vi "Main Program Oringin.vi"() -> ()   [LabVIEW 2019]
uses:
  <vilib>/rvi/interface/nirviMethod/nirviMethod.xnode
  <vilib>/rvi/interface/nirviReadWriteControl/nirviReadWriteControl.xnode
  <vilib>/FPGAPlugInAG/Dynamic/niLvFpga_Run_Dynamic.vi
  <vilib>/FPGAPlugInAG/Dynamic/niLvFpga_Abort_Dynamic.vi
  <vilib>/platform/TimedLoop/XDataNode/XDataNode.xnode
  <vilib>/Platform/TimedLoop/XDataNode/nitl_modes.ctl
  <vilib>/Platform/TimedLoop/XDataNode/XDNodeRunTimeDep.lvlib
  <vilib>/Platform/TimedLoop/XDataNode/wakeup.ctl
  <vilib>/Platform/TimedLoop/XDataNode/timing_clust.ctl
  <vilib>/Utility/error.llb/Error Cluster From Error Code.vi
  <vilib>/rvi/interface/Simulation/niFpgaSimulationCallBeginRW.vi
  <vilib>/rvi/errors/niLvFpgaAdjustHostInterfaceError.vi
  NiFpgaLv.dll
  <vilib>/rvi/interface/nirviOpenFPGA/nirviOpenFPGA.xnode
  FPGA Bitfiles/fpgaproject_FPGATarget_Fpga_-EhYRlmx2hw.lvbitx
  Fpga.vi
  <vilib>/FPGAPlugInAG/Dynamic/niLvFpga_StartFifo_Dynamic.vi
  <vilib>/rvi/errors/niLvFpgaMergeErrorWithErrorCode.vi
  <vilib>/FPGAPlugInAG/cRIO-9065/niLvFpga_Open_cRIO-9065.vi
  <vilib>/rvi/interface/common/dynamic/niFpgaDynamicAddResources.vi
panel:
  out "error out 3":errorcluster
  in  "string":string
  in  "Vlotage In":fxp<+/-,20,5>
  out "Real Period":u32[](array[numeric])
  out "Set period":i64[](array[numeric])
  out "Real Period":u32
  out "Voltage Out":fxp<+/-,20,5>
  out "size(s)":i32[](array[numeric])
  in  "Period":i64
  out "Encoder Position":dbl format="%#_8g"
  in  "Position Reset":bool
  out "data":string[][](array[string])
  out "速率":dbl
  out "error out 2":errorcluster
  out "error out":errorcluster
  in  "stop":bool
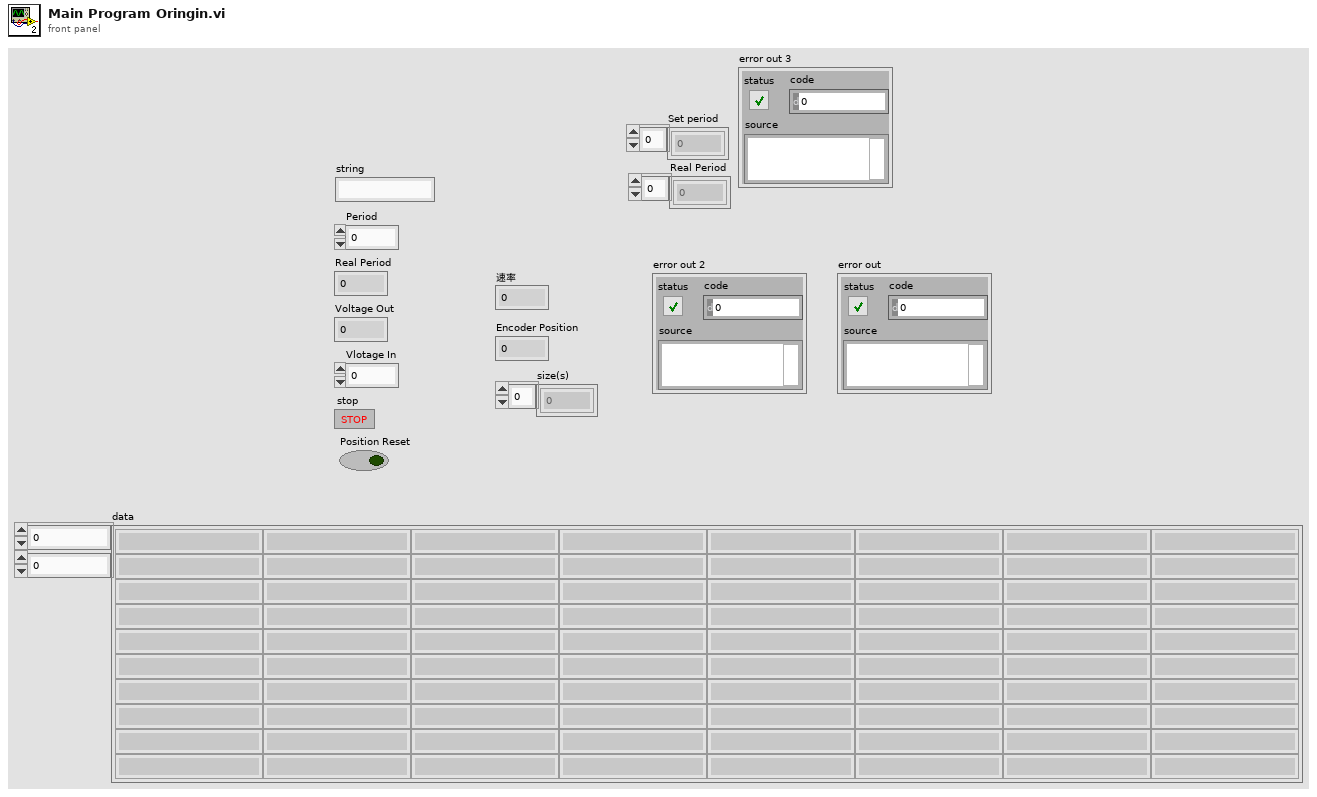
[diagram p1: front panel]
types:
  T1 = enum16{"open", "replace", "create", "open or create", "replace or create", "replace or create with confirmation"}
  T2 = typedef "XDNodeRunTimeDep.lvlib/timing_clust.ctl" = cluster{"Expected End [f-1]":u64, "Actual End [f-1]":u64, "Finished Late? [f-1]":bool, "Expected End [i-1]":u64, "Actual End [i-1]":u64, "Finished Late? [i-1]":bool, "Expected Start [i]":u64, "Actual Start [i]":u64, "Expected Start [f]":u64, "Actual Start [f]":u64, "Source Name":string, "Structure Name":string, "Period":i64, "Deadline":i64, "Offset":i64, "Start":i64, "Priority":i32, "Timeout":i32, "Mode":T3, "Wakeup Reason":T4, "Error":errorcluster, "Source Type":string, "Secondary Source Type":string, "Global End Time":u64, "Global Start Time":u64, "Frame Duration":u64, "Iteration Duration":u64, "Assigned CPU":i32, "I/O Scan Engine Mode":u32}
  T3 = typedef "XDNodeRunTimeDep.lvlib/nitl_modes.ctl" = enum32{"No Change", "Process missed periods, maintain original phase", "Discard missed periods, maintain original phase", "Process missed periods, ignore original phase", "Discard missed periods, ignore original phase"}
  T4 = typedef "XDNodeRunTimeDep.lvlib/wakeup.ctl" = enum32{"Normal", "Aborted", "Asynchronous wakeup", "Timing source error", "Timed loop error", "Timeout"}
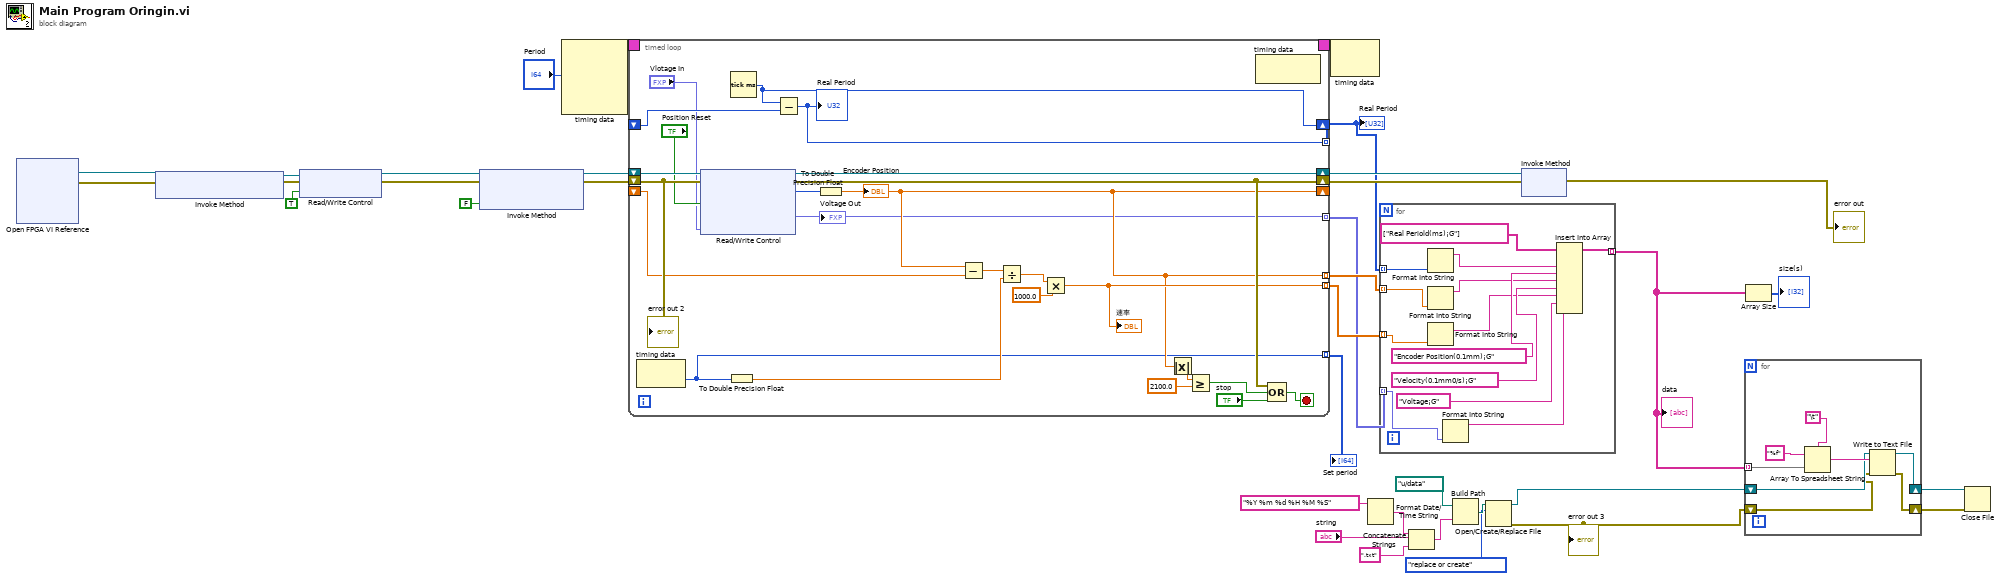
[diagram p0: block diagram]
diagram:
  n1 = xnode "Open FPGA VI Reference"() -> ("FPGA VI Reference Out"=w16:refnum<k20>, "error out"=w15:errorcluster)  [unwired: 2 in]
  n2 = xnode "Invoke Method"("FPGA VI Reference In"=w16, "error in"=w15) -> ("FPGA VI Reference Out"=w25:refnum<k20>, "error out"=w24:errorcluster)
  n3 = xnode "Read/Write Control"("FPGA VI Reference In"=w25, "error in"=w24, "Position Reset"=TRUE) -> ("FPGA VI Reference Out"=w33:refnum<k20>, "error out"=w32:errorcluster)
  n4 = xnode "Invoke Method"("FPGA VI Reference In"=w33, "error in"=w32, "Wait Until Done (F)"=FALSE) -> ("FPGA VI Reference Out"=w12:refnum<k20>, "error out"=w11:errorcluster)
  n5 = node-c288("Period") -> (w28:T2)  [unwired: 3 in]
  n6 = timed-loop {
    shift-right: [w57] -> w35
    shift-left: w12 -> [w55]
    shift-right: [w50] -> w34
    shift-left: w11 -> [w58]
    timing: w28 -> [_]
    timing-out: [_] -> w27
    shift-right: [w42] -> _
    shift-left: _ -> [w56]
    tunnel: [w42] -> w23 mode=indexing
    tunnel: [w44] -> w21 mode=indexing
    tunnel: [w41] -> w17 mode=indexing
    tunnel: [w40] -> w14 mode=indexing
    shift-right: [w38] -> _
    shift-left: _ -> [w39]
    tunnel: [w37] -> w13 mode=indexing
    stop <- w52 stop-if-true
    n7 = node-c288() -> (w40:i64)  [unwired: 1 in]
    n8 = xnode "Read/Write Control"("FPGA VI Reference In"=w55, "error in"=w58, "Position Reset"="Position Reset", "Voltage In"="Vlotage In") -> ("FPGA VI Reference Out"=w57:refnum<k20>, "error out"=w50:errorcluster, "Position (Counts)"=w47:i32, "Voltage Out"=w41:fxp<+/-,20,5>)
    "Voltage Out" <- w41
    n9 = To Double Precision Float(number=w40) -> (double precision float=w46:dbl)
    n10 = Tick Count (ms)() -> (millisecond timer value=w38:u32)
    n11 = Subtract(x=w38, y=w39) -> (x-y=w37:u32)
    "Real Period" <- w37
    n12 = To Double Precision Float(number=w47) -> (double precision float=w42:dbl)
    "Encoder Position" <- w42
    n13 = Subtract(x=w42, y=w56) -> (x-y=w59:dbl)
    n14 = Divide(x=w59, y=w46) -> (x/y=w45:dbl)
    n15 = Multiply(x=w45, y=1000.0) -> (x*y=w44:dbl)
    "速率" <- w44
    n16 = Absolute Value(x=w42) -> (abs(x)=w43:dbl)
    n17 = Greater Or Equal?(x=w43, y=2100.0) -> (x >= y?=w49:bool)
    n18 = node-c288() -> ()  [unwired: 1 in, 1 out]
    n19 = Compound Arithmetic op=OR(w50, w49, "stop") -> (w52:bool)
    "error out 2" <- w58
  }
  "Set period" <- w14
  "Real Period" <- w13
  n20 = node-c288(w27) -> ()  [unwired: 1 out]
  n21 = Format Date/Time String(time format string (%c)="%Y %m %d %H %M %S") -> (date/time string=w8:string)  [unwired: 2 in]
  n22 = for {
    tunnel: [w73] -> w19 mode=indexing
    tunnel: w23 -> [w70] mode=indexing
    tunnel: w21 -> [w72] mode=indexing
    tunnel: w17 -> [w65] mode=indexing
    tunnel: w13 -> [w63] mode=indexing
    n23 = Format Into String(w63) -> (resulting string=w68:string)  [unwired: 3 in, 1 out]
    n24 = Format Into String(w70) -> (resulting string=w69:string)  [unwired: 3 in, 1 out]
    n25 = Format Into String(w72) -> (resulting string=w71:string)  [unwired: 3 in, 1 out]
    n26 = Format Into String(w65) -> (resulting string=w64:string)  [unwired: 3 in, 1 out]
    n27 = Insert Into Array(array=string[] ["Real Periold(ms)¡G"], new element #1=w68, new element #2="Encoder Position(0.1mm)¡G", new element #3=w69, new element #4="Velocity(0.1mm0/s)¡G", new element #5=w71, new element #6="Voltage¡G", new element #7=w64) -> (w73:string[])  [unwired: 1 in]
  }
  "data" <- w19
  n28 = Concatenate Strings(w8, "string", ".txt" ("element")) -> (w7:string)
  n29 = Build Path(base path=path "u:/data", name or relative path=w7) -> (appended path=w9:path)
  n30 = Open/Create/Replace File(file path (use dialog)=w9, operation (0:open)=T1."replace or create") -> (refnum out=w4:refnum<file>, error out=w3:errorcluster)  [unwired: 4 in, 1 out]
  "error out 3" <- w3
  n31 = xnode "Invoke Method"("FPGA VI Reference In"=w35, "error in"=w34) -> ("error out"=→"error out":errorcluster)  [unwired: 1 out]
  n32 = for {
    shift-right: [w77] -> w29
    shift-left: w4 -> [w80]
    shift-right: [w78] -> w30
    shift-left: w3 -> [w79]
    tunnel: w19 -> [w76] mode=indexing
    n33 = Array To Spreadsheet String(delimiter (Tab)="\t", array=w76, 3:"%f" ("format string")) -> (spreadsheet string=w81:string)
    n34 = Write to Text File(file (use dialog)=w80, text=w81, error in=w79) -> (refnum out=w77:refnum<file>, error out=w78:errorcluster)  [unwired: 1 in, 1 out]
  }
  n35 = Array Size(array=w19) -> (size(s)=→"size(s)":i32[])
  n36 = Close File(refnum=w29, error in=w30) -> ()  [unwired: 2 out]
